vi "safetiptrigger.vi"(11 "triggered":bool) -> ()   [LabVIEW 2017, in "HapticSTM.lvlib"]
doc: "extern \"C\" __declspec(dllexport) void safetiptrigger(bool triggered);"
uses:
  HapticSTM.lvlib
  <userlib>/HapticSTM/HapticSTM.dll
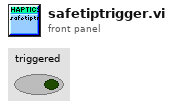
[diagram p1: front panel]
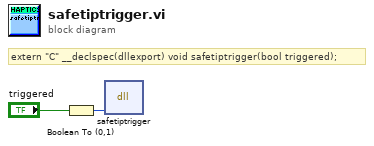
[diagram p0: block diagram]
diagram:
  # "extern \"C\" __declspec(dllexport) void safetiptrigger(bool triggered);"
  n1 = Boolean To (0,1)(Boolean="triggered") -> (0, 1=w1:i16)
  n2 = dll-call lib="C:/Program Files/National Instruments/LabVIEW 2019/user.lib/HapticSTM/HapticSTM.*" fn="safetiptrigger"("triggered"=w1) -> ()  [unwired: 5 in, 2 out]
